vi "Load.vi"(8 "error in":errorcluster, 10 "Source":string, 11 "gRPC XNET Read Raw CAN Frame Strategy in":refnum<class "gRPC XNET Read Raw CAN Frame Strategy.lvclass">) -> (0 "error out":errorcluster, 3 "gRPC XNET Read Raw CAN Frame Strategy out":refnum<class "gRPC XNET Read Raw CAN Frame Strategy.lvclass">)   [LabVIEW 2024, in "gRPC XNET Read Raw CAN Frame Strategy.lvclass"]
uses:
  gRPC XNET Read Raw CAN Frame Strategy.lvclass
  gRPC XNET Read Raw CAN Frame Strategy.lvclass/gRPC XNET Read Raw CAN Frame Strategy.ctl
  Source/Config from JSON/Config from JSON.lvclass
  D:/git/HAL/Source/Config from JSON/Config from JSON.lvclass
  D:/git/HAL/Source/Interfaces/IConfiguration/IConfiguration.lvclass
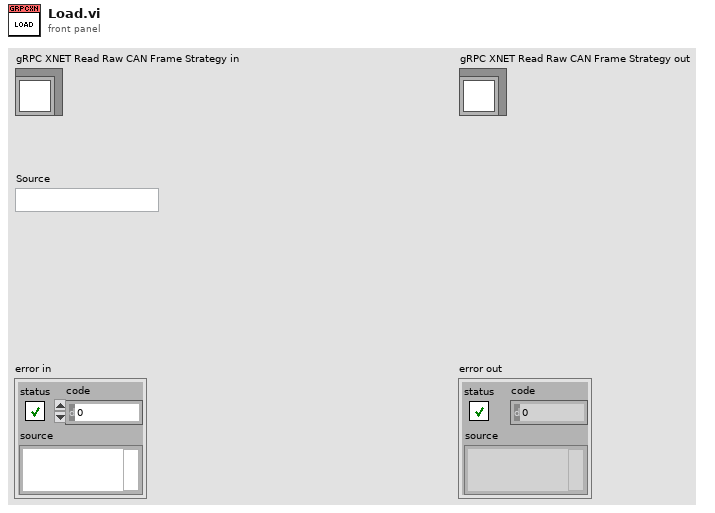
[diagram p1: front panel]
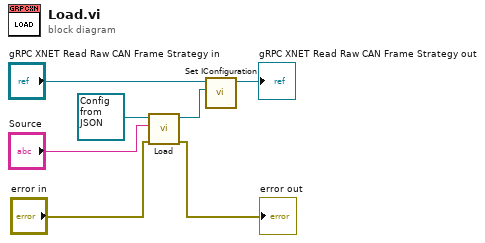
[diagram p0: block diagram]
diagram:
  n1 = call-dynamic "Load.vi"("error in"="error in", "Source"="Source", "Config From JSON in"=refnum<class "Config from JSON.lvclass"> refnum ("Config from JSON.lvclass")) -> ("error out"=→"error out":errorcluster, "Config From JSON out"=w1:refnum<class "Config from JSON.lvclass">)  [unwired: 7 in]
  n2 = call-dynamic "Set IConfiguration.vi"("IConfiguration"=w1, "gRPC XNET Read Raw CAN Frame Strategy in"="gRPC XNET Read Raw CAN Frame Strategy in") -> ("gRPC XNET Read Raw CAN Frame Strategy out"=→"gRPC XNET Read Raw CAN Frame Strategy out":refnum<class "gRPC XNET Read Raw CAN Frame Strategy.lvclass">)  [unwired: 9 in]
